vi "SetControlVIandRun.vi"(10 "Controlling VI path":path=path "", 11 "appended path":path) -> (3 "Sub VI out":refnum<vi>)   [LabVIEW 2022 SP3]
panel:
  out "error out":errorcluster
  in  "error in (no error)":errorcluster
  out "Controller VI Path Set":path
  out "Labels":string[](array[string])
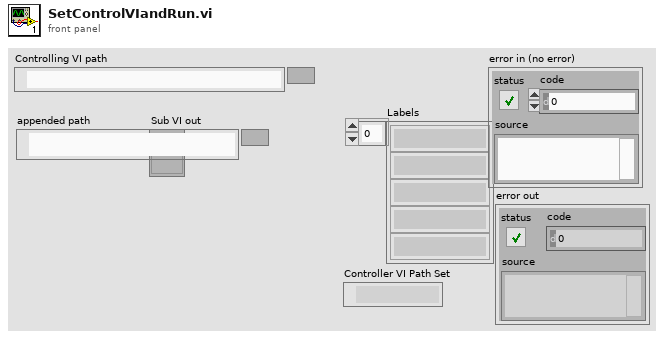
[diagram p1: front panel]
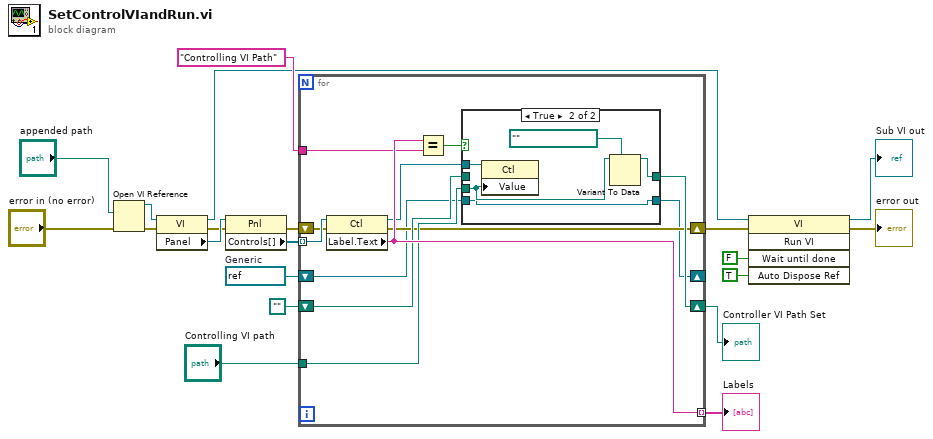
[diagram p0: block diagram]
diagram:
  w1 = refnum<vi> refnum  # Generic
  n1 = Open VI Reference(vi path="appended path", error in (no error)="error in (no error)") -> (vi reference=w9:refnum<vi>, error out=w4:errorcluster)  [unwired: 4 in]
  n2 = property class="VI"(reference=w9, error in=w4) -> (reference out=w8:refnum<vi>, error out=w5:errorcluster, "Panel"=w20:refnum<vi>)
  n3 = property class="Pnl"(reference=w20, error in=w5) -> (error out=w6:errorcluster, "Controls[]"=w18:refnum<vi>[])  [unwired: 1 out]
  n4 = for {
    tunnel: w18 -> [w32] mode=indexing
    tunnel: [w31] -> w17 mode=indexing
    shift-right: [w28] -> w15
    shift-left: path "" -> [w27]
    tunnel: "Controlling VI path" -> [w26]
    tunnel: "Controlling VI Path" -> [w25]
    shift-right: [w24] -> w10
    shift-left: w6 -> [w23]
    shift-right: [w22] -> _
    shift-left: w1 -> [w21]
    n5 = property class="Ctl"(reference=w32, error in=w23) -> (reference out=w30:refnum<vi>, error out=w24:errorcluster, "Label.Text"=w31:string)
    n6 = Equal?(x=w31, y=w25) -> (x = y?=w29:bool)
    n7 = case shown="True" w29 {
      tunnel: w30 -> [_ w39]
      tunnel: [w34 w37] -> w28
      tunnel: w27 -> [w34 _]
      tunnel: w26 -> [_ w36]
      tunnel: [w33 w35] -> w22
      tunnel: w21 -> [w33 w35]
      frame False {
      }
      frame True {
        n8 = property class="Ctl"(reference=w39, "Value"=w36) -> ()  [unwired: 1 in, 2 out]
        n9 = Variant To Data(type=path "", Variant=w36) -> (data=w37:path)  [unwired: 1 in, 1 out]
      }
    }
  }
  "Labels" <- w17
  "Controller VI Path Set" <- w15
  n10 = invoke class="VI" method="Run VI"(reference=w8, error in=w10, "Wait until done"=FALSE ("Wait Until Done"), "Auto Dispose Ref"=TRUE ("Auto Dispose Reference")) -> (reference out=→"Sub VI out":refnum<vi>, error out=→"error out":errorcluster)  [unwired: 1 in, 3 out]
